vi "ROI entry-Actions on all ROI cleared.vi"(11 "No ROIs (T)":bool=TRUE) -> ()   [LabVIEW 2020]
uses:
  Typedefs/ROI management FG states.ctl
  ROI Entry screen/Typedefs/ROI input mode.ctl
  ROI Entry screen/Globals/gl_ROI Entry UI globals.vi
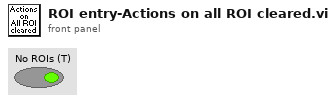
[diagram p1: front panel]
types:
  T1 = typedef "ROI management FG states.ctl" = enum16{"Read", "Write", "Write-from dataset", "Clear Last", "Clear All", "Delete ROI", "Update ROIs time", "Reload last ROI set", "Modify ROI Parameters", "Offset all ROI", "Offset visible ROI", "Modify Dwell Time", "Modify Laser Power"}
  T2 = enum8{"Enabled", "Disabled", "Disabled and Grayed Out"}
  T3 = typedef "ROI input mode.ctl" = enum16{"Unspecified", "Point-Line-Plane", "Volume"}
  T4 = typedef "IMAQ Image.ctl" = refnum<image>
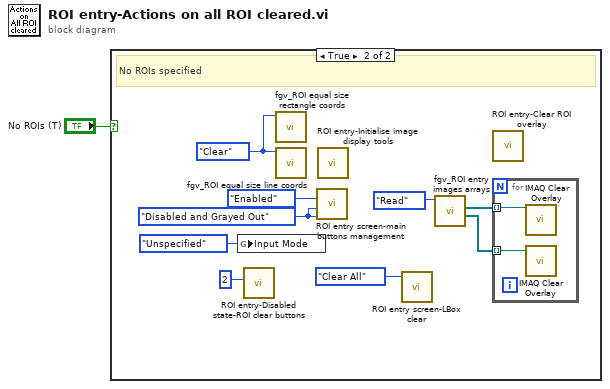
[diagram p0: block diagram]
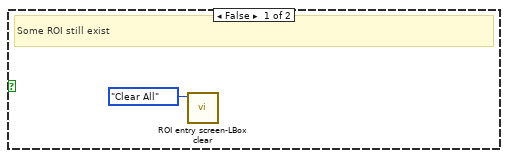
[diagram p2: hidden frame]
diagram:
  n1 = case shown="True" "No ROIs (T)" {
    frame False {
      # "Some ROI still exist"
      n2 = call "ROI entry screen-LBox clear.vi"("Function"=ROI_management_FG_states."Clear All") -> ()  [unwired: 10 in, 1 out]
    }
    frame True {
      w4 = enum16{"Intialize", "Write", "Read", "Clear"}."Clear" ("Function")
      w11 = T2."Disabled and Grayed Out" ("Disabled")
      # "No ROIs specified"
      n3 = global write "gl_ROI Entry UI globals.vi" "Input Mode"(ROI_input_mode."Unspecified" ("Input Mode")) -> ()
      n4 = call "ROI entry-Disabled state-ROI clear buttons.vi"("State"=2) -> ()  [unwired: 10 in, 1 out]
      n5 = call "fgv_ROI equal size rectangle coords.vi"("Function"=w4) -> ()  [unwired: 9 in, 2 out]
      n6 = call "fgv_ROI equal size line coords.vi"("Function"=w4) -> ()  [unwired: 9 in, 2 out]
      n7 = call "ROI entry screen-main buttons management.vi"("Imaging button disabled?"=w11, "Acquisition button disabled?"=w11, "Done button disabled?"=T2."Enabled") -> ()  [unwired: 9 in]
      n8 = call "ROI entry-Initialise image display tools.vi"() -> ()  [unwired: 11 in, 1 out]
      n9 = call "ROI entry screen-LBox clear.vi"("Function"=ROI_management_FG_states."Clear All") -> ()  [unwired: 10 in, 1 out]
      n10 = call "fgv_ROI entry images arrays.vi"("Function"=enum16{"Intialize", "Write", "Read", "Clear"}."Read") -> ("GreenImageArray"=w7:T4[], "RedImageArray"=w6:T4[])  [unwired: 8 in, 1 out]
      n11 = call "ROI entry-Clear ROI overlay.vi"() -> ()  [unwired: 10 in, 2 out]
      n12 = for {
        tunnel: w6 -> [w13] mode=indexing
        tunnel: w7 -> [w12] mode=indexing
        n13 = call "IMAQ Clear Overlay"("Image"=w13) -> ()  [unwired: 9 in, 2 out]
        n14 = call "IMAQ Clear Overlay"("Image"=w12) -> ()  [unwired: 9 in, 2 out]
      }
    }
  }
